vi "get_position_robust (SubVI).vi"(8 "error in (no error)":errorcluster, 9 "motor":i32, 10 "deviceKey":string, 11 ".NET Refnum in":refnum<k24>) -> (0 "error out":errorcluster, 1 "position":i32, 2 "GetPosition":bool, 3 ".NET Refnum out":refnum<k24>)   [LabVIEW 2016]
uses:
  C:/Users/UsphereLab/Documents/GitHub/Optlev/LabView Code/Examples/Tilt Stage/CmdLib.dll
  Examples/Tilt Stage/CmdLib.dll
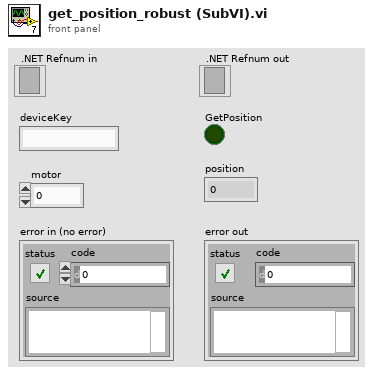
[diagram p1: front panel]
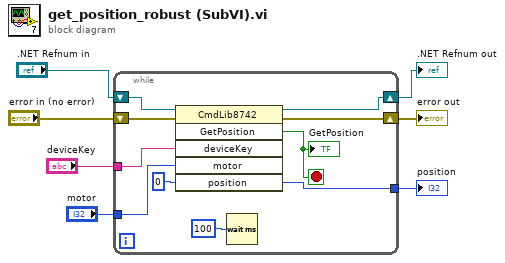
[diagram p0: block diagram]
diagram:
  n1 = while {
    tunnel: "deviceKey" -> [w13]
    shift-right: [w14] -> w5
    shift-left: "error in (no error)" -> [w11]
    shift-right: [w15] -> w6
    shift-left: ".NET Refnum in" -> [w10]
    tunnel: "motor" -> [w12]
    tunnel: [w17] -> w7
    stop <- w9 stop-if-true
    n2 = invoke class="CmdLib8742" method="GetPosition"(reference=w10, error in=w11, "deviceKey"=w13, "motor"=w12, "position"=0) -> (reference out=w15:refnum<k24>, error out=w14:errorcluster, "GetPosition"=w9:bool, "position"=w17:i32)  [unwired: 1 in, 2 out]
    "GetPosition" <- w9
    n3 = Wait (ms)(milliseconds to wait=u32 100) -> ()  [unwired: 1 out]
  }
  "position" <- w7
  ".NET Refnum out" <- w6
  "error out" <- w5
